vi "ZK蠕动泵频率参数写入.vi"(7 "是否启用通讯通知":bool, 8 "error in (no error)":errorcluster, 9 "蠕动泵最小频率":i32, 10 "蠕动泵最大频率":i32, 11 "Slave ID":T1) -> (0 "error out":errorcluster)   [LabVIEW 2016, in "质控单元V4.lvlib"]
uses:
  <vilib>/Plasmionique/MB Master/MB_Master/MB_Master.lvclass
  <vilib>/Plasmionique/MB Master/MB Master.lvlib
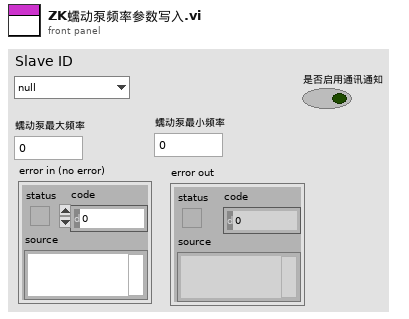
[diagram p1: front panel]
types:
  T1 = typedef "质控单元V4.lvlib/质控slave id.ctl" = enum16{"null", "氨氮", "总磷", "总氮", "CODMn", "CODCr"}
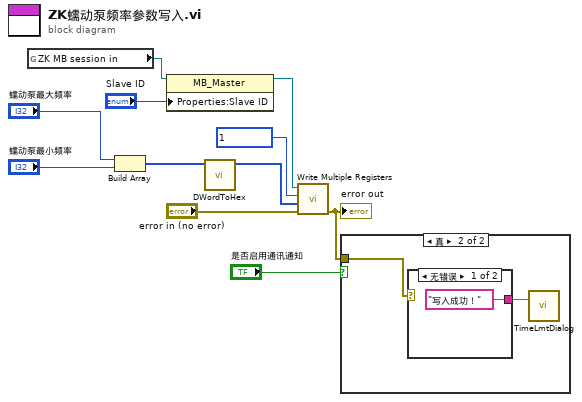
[diagram p0: block diagram]
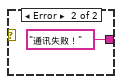
[diagram p3: hidden frame]
diagram:
  n1 = global read "ZK非断电保存全局变量.vi" "ZK MB session in"() -> (w10:refnum<class "MB_Master.lvclass">)
  n2 = Build Array("蠕动泵最大频率", "蠕动泵最小频率") -> (w4:i32[])
  n3 = property class="MB_Master"(reference=w10, "Properties:Slave ID"="Slave ID") -> (reference out=w8:refnum<class "MB_Master.lvclass">)  [unwired: 1 in, 1 out]
  n4 = call "DWordToHex.vi"("DWORD"=w4) -> ("数组"=w3:u16[])  [unwired: 10 in]
  n5 = call <vilib>:"Write Multiple Registers.vi"("error in (no error)"="error in (no error)", "values"=w3, "starting address"=u16 1, "MB session in"=w8) -> ("error out"=w1:errorcluster)  [unwired: 6 in, 1 out]
  "error out" <- w1
  n6 = case shown="真" "是否启用通讯通知" {
    tunnel: w1 -> [_ w13]
    frame False {
    }
    frame True {
      n7 = case shown="无错误" w13 {
        tunnel: ["写入成功！" "通讯失败！"] -> w12
        frame No Error {
        }
        frame Error {
        }
      }
      n8 = call "TimeLmtDialog.vi"("Infoin"=w12) -> ()  [unwired: 11 in]
    }
  }
